vi "Read Registers.vi"(6 "Register Size":T1, 7 "Slave Address":u8, 8 "Error In":errorcluster, 9 "Count":i32, 10 "Register":u32, 11 "I2C In":refnum<class "I2C.lvclass">) -> (0 "Error Out":errorcluster, 2 "Values":u8[](array[numeric]), 3 "I2C Out":refnum<class "I2C.lvclass">)   [LabVIEW 2020, in "lv_i2c_hal.lvlib" / "I2C.lvclass"]
uses:
  I2C.lvclass
  Register Address Size.ctl
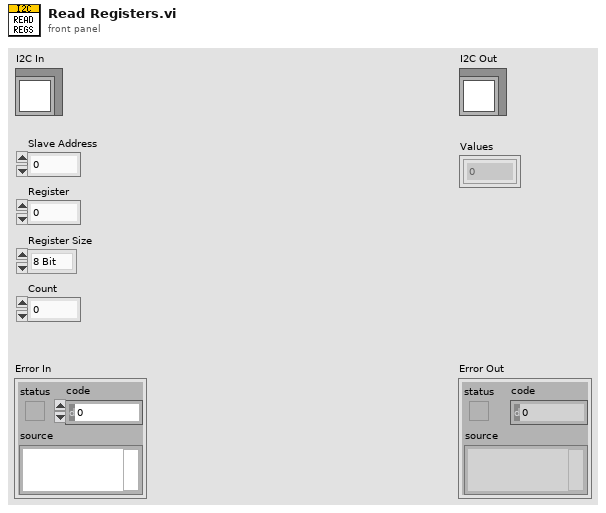
[diagram p1: front panel]
types:
  T1 = typedef "lv_i2c_hal.lvlib/I2C.lvclass/Register Address Size.ctl" = enum16{"8 Bit", "16 Bit", "24 Bit", "32 Bit"}
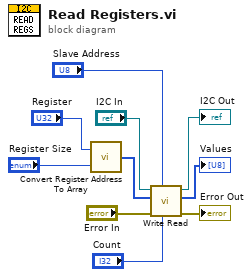
[diagram p0: block diagram]
diagram:
  n1 = call "Convert Register Address To Array.vi"("Register Address Size"="Register Size", "Register"="Register") -> ("Register Address Array"=w7:u8[])
  n2 = call-dynamic "Write Read.vi"("Count"="Count", "Slave Address"="Slave Address", "Error In"="Error In", "Data In"=w7, "I2C In"="I2C In") -> ("Error Out"=→"Error Out":errorcluster, "Data Out"=→"Values":u8[], "I2C Out"=→"I2C Out":refnum<class "I2C.lvclass">)  [unwired: 4 in]
